vi "ReadClusterFromFile.vi"(9 "Name":string, 10 "Cluster in":refnum<vi>, 11 "ConfigIn":T1) -> (3 "ConfigOut":T1)   [LabVIEW 2015]
uses:
  <vilib>/Utility/config.llb/Config Data RefNum.ctl
  <vilib>/Utility/config.llb/NI_LVConfig.lvlib
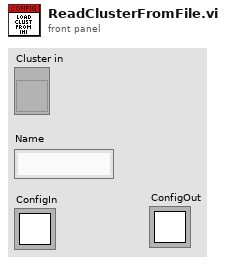
[diagram p1: front panel]
types:
  T1 = typedef "NI_LVConfig.lvlib/Config Data RefNum.ctl" = refnum<k1>
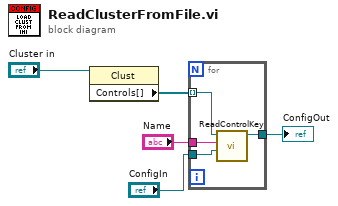
[diagram p0: block diagram]
diagram:
  n1 = property class="Clust"(reference="Cluster in") -> ("Controls[]"=w3:refnum<vi>[])  [unwired: 1 in, 2 out]
  n2 = for {
    tunnel: w3 -> [w9] mode=indexing
    tunnel: "ConfigIn" -> [w8]
    tunnel: "Name" -> [w7]
    tunnel: [w6] -> w1
    n3 = call "ReadControlKey.vi"("ConfigFile"=w8, "section"=w7, "Control in"=w9) -> ("ConfigFile out"=w6:T1)  [unwired: 8 in]
  }
  "ConfigOut" <- w1
